vi "Wait On Occurence.vi"(8 "error in":errorcluster, 10 "ms timeout (-1)":i32=-1, 11 "occurrence in":refnum<k4>) -> (0 "error out":errorcluster)   [LabVIEW 2019]
uses:
  <vilib>/Utility/error.llb/Error Cluster From Error Code.vi
  grpc-lvsupport.lvlib
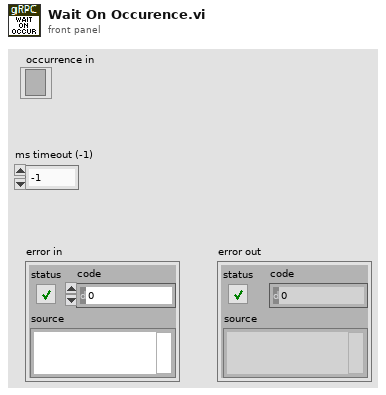
[diagram p1: front panel]
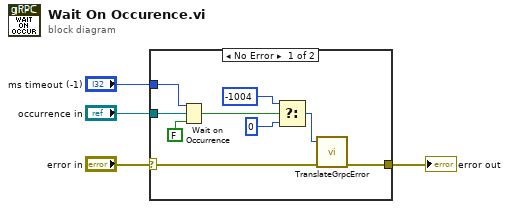
[diagram p0: block diagram]
diagram:
  n1 = case shown="No Error" "error in" {
    selector: "error in" -> [w13 w14]
    tunnel: [w11 w14] -> w3
    tunnel: "occurrence in" -> [w12 _]
    tunnel: "ms timeout (-1)" -> [w6 _]
    frame No Error {
      n2 = Wait on Occurrence(1:FALSE ("ignore previous (T)"), 2:w12, 3:w6) -> (0:w10:bool)
      n3 = Select(t=-1004 ("Error Code"), s=w10, f=0 ("Error Code")) -> (s? t:f=w7:i32)
      n4 = call "TranslateGrpcError.vi"("error in"=w13, "Error Code"=w7) -> ("error out"=w11:errorcluster)  [unwired: 9 in]
    }
    frame Error {
    }
  }
  "error out" <- w3
